vi "Eval y=f(x1,x2).vi"(0 "Start":dbl[](array[numeric])=[0.0, 0.0] format="%.2f", 1 "number of points":u32=25, 2 "End":dbl[](array[numeric])=[1.0, 1.0] format="%.2f", 3 "formula":string, 4 "Variables":string[](array[string])=["x1", "x2"]) -> (5 "X1 Values":dbl[](array[numeric]) format="%.2f", 6 "X2 Values":dbl[](array[numeric]) format="%.2f", 7 "Y Values":dbl[][](array[numeric]) format="%.2f", 8 "ticks":u32, 9 "error":i32)   [LabVIEW 2017, in "NI_Gmath.lvlib"]
doc: "Calculates a 2D array of function values defined on a grid."
uses:
  <vilib>/gmath/NI_Gmath.lvlib
panel:
  # "Example:\n\n number of points: 25 \n Start: 0.0 and 0.0\n End: 1.0 and 1.0\n formula: 7*sin(x1)-cos(3*x2) \n Variables: x1 and x2"
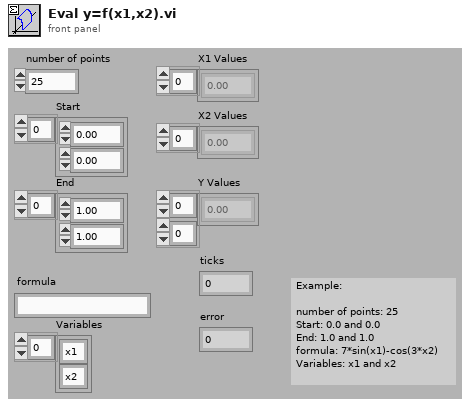
[diagram p1: front panel]
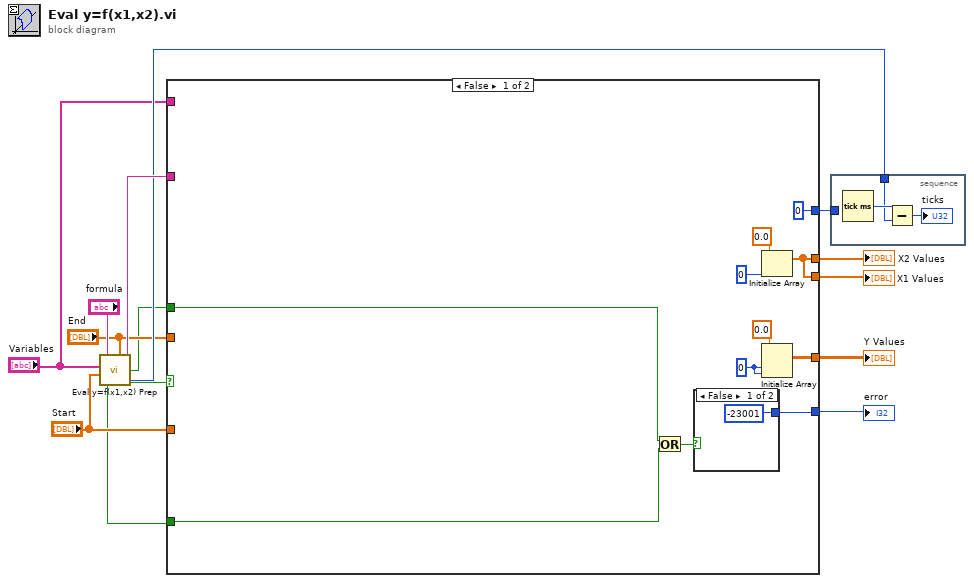
[diagram p0: block diagram]
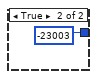
[diagram p2: hidden frame]
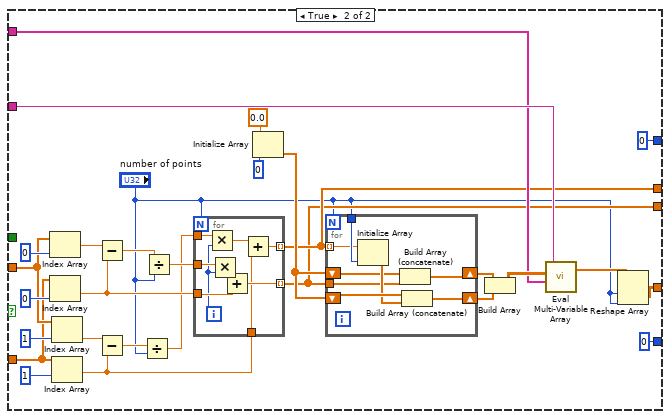
[diagram p3: hidden frame]
diagram:
  n1 = call <vilib>:"Eval y=f(x1,x2) Prep.vi"("End"="End", "Start"="Start", "Variables"="Variables", "formula"="formula") -> ("time [msec]"=w12:u32, "error (general)"=w6:bool, "error situation 1"=w1:bool, "formula copy"=w13:string, "error situation 2"=w3:bool)
  n2 = case shown="False" w6 {
    tunnel: [0 0] -> w14
    tunnel: w13 -> [_ w37]
    tunnel: "Variables" -> [_ w34]
    tunnel: [w22 w36] -> w11
    tunnel: [w21 0] -> w9
    tunnel: "End" -> [_ w32]
    tunnel: "Start" -> [_ w31]
    tunnel: w1 -> [w17 _]
    tunnel: [w18 w30] -> w5
    tunnel: [w18 w29] -> w4
    tunnel: w3 -> [w15 _]
    frame False {
      w23 = 0
      n3 = Or(x=w17, y=w15) -> (x .or. y?=w16:bool)
      n4 = case shown="False" w16 {
        tunnel: [-23001 -23003] -> w21
        frame False {
        }
        frame True {
        }
      }
      n5 = Initialize Array(0.0, 0) -> (w18:dbl[])
      n6 = Initialize Array(0.0, w23, w23) -> (w22:dbl[][])
    }
    frame True {
      n7 = Index Array(array=w32, index=0) -> (element=w52:dbl)
      n8 = Index Array(array=w31, index=0) -> (element=w53:dbl)
      n9 = Index Array(array=w32, index=1) -> (element=w54:dbl)
      n10 = Index Array(array=w31, index=1) -> (element=w55:dbl)
      n11 = Subtract(x=w52, y=w53) -> (x-y=w38:dbl)
      n12 = Subtract(x=w54, y=w55) -> (x-y=w45:dbl)
      n13 = Divide(x=w45, y="number of points") -> (x/y=w46:dbl)
      n14 = Divide(x=w38, y="number of points") -> (x/y=w47:dbl)
      n15 = for {
        N: "number of points" -> [_]
        tunnel: w47 -> [w65]
        tunnel: w53 -> [w63]
        tunnel: [w62] -> w29 mode=indexing
        tunnel: w46 -> [w61]
        tunnel: w55 -> [w58]
        tunnel: [w57] -> w30 mode=indexing
        i -> [w60]
        n16 = Multiply(x=w61, y=w60) -> (x*y=w59:dbl)
        n17 = Multiply(x=w65, y=w60) -> (x*y=w64:dbl)
        n18 = Add(x=w64, y=w63) -> (x+y=w62:dbl)
        n19 = Add(x=w59, y=w58) -> (x+y=w57:dbl)
      }
      n20 = Initialize Array(0.0, 0) -> (w42:dbl[])
      n21 = for {
        N: "number of points" -> [_]
        tunnel: "number of points" -> [w73]
        tunnel: w30 -> [w72] mode=indexing
        shift-right: [w70] -> w44
        shift-left: w42 -> [w71]
        shift-right: [w68] -> w43
        shift-left: w42 -> [w67]
        tunnel: w29 -> [w66]
        n22 = Initialize Array(w72, w73) -> (w69:dbl[])
        n23 = Build Array (concatenate)(w67, w66) -> (w68:dbl[])
        n24 = Build Array (concatenate)(w71, w69) -> (w70:dbl[])
      }
      n25 = Build Array(w43, w44) -> (w35:dbl[][])
      n26 = call <vilib>:"Eval Multi-Variable Array.vi"("Variables"=w34, "X Values"=w35, "formula"=w37) -> ("Y Values"=w39:dbl[])  [unwired: 1 in, 1 out]
      n27 = Reshape Array(w39, "number of points", "number of points") -> (w36:dbl[][])
    }
  }
  "Y Values" <- w11
  "error" <- w9
  "X1 Values" <- w4
  "X2 Values" <- w5
  n28 = stacked-sequence {
    tunnel: w14 -> [_]
    tunnel: w12 -> [w74]
    frame #0 {
      n29 = Tick Count (ms)() -> (millisecond timer value=w76:u32)
      n30 = Subtract(x=w76, y=w74) -> (x-y=→"ticks":u32)
    }
  }
